vi "functional global counter 2.vi"() -> ()   [LabVIEW 2010]
uses:
  Functional Global Command.ctl
panel:
  out "카운트 2":i32
  out "진행 중 합계":i32
  out "전체 카운트":i32
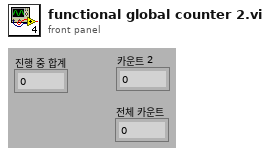
[diagram p1: front panel]
types:
  T1 = typedef "Functional Global Command.ctl" = enum16{"리셋", "증가", "카운트 가져오기"}
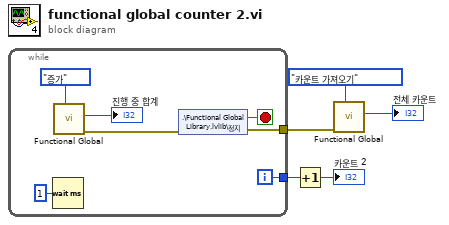
[diagram p0: block diagram]
diagram:
  n1 = while {
    tunnel: [w12] -> w5
    tunnel: [w11] -> w3
    i -> [w12]
    stop <- w6 stop-if-true
    n2 = Wait (ms)(milliseconds to wait=u32 1) -> ()  [unwired: 1 out]
    n3 = call "Functional Global.vi"("명령"=Functional_Global_Command."증가" ("Command")) -> ("에러 출력"=w8:errorcluster, "카운트"=→"진행 중 합계":i32)  [unwired: 9 in]
    n4 = shared-variable ".\\Functional Global Library.lvlib\\정지"(error in=w8) -> (w6:bool, error out=w11:errorcluster)
  }
  n5 = Increment(x=w5) -> (x+1=→"카운트 2":i32)
  n6 = call "Functional Global.vi"("명령"=Functional_Global_Command."카운트 가져오기" ("Command"), "에러 입력 (에러 없음)"=w3) -> ("카운트"=→"전체 카운트":i32)  [unwired: 8 in, 1 out]
